vi "NovaTech409A_FreqPowPhase.vi"(2 "error in (no error)":errorcluster, 3 "Channel (0-3)":u8 max=3, 4 "Phase":u16 max=16383, 5 "Power":u16 max=1023, 6 "Freq":dbl=10.0 min=0.0 max=171.1276031, 7 "VISA resource name":refnum<visa-resource-name>="COM1") -> (0 "error out":errorcluster, 1 "VISA resource name out":refnum<visa-resource-name>="COM1")   [LabVIEW 2013, in "Novatech 409A.lvlib"]
uses:
  Novatech 409A.lvlib
panel:
  out "resulting string 3":string="P0 00000\n"
  out "read buffer 3":string
  out "resulting string 2":string="V0 0000\n"
  out "resulting string":string="F0 010.0000000\n"
  out "read buffer 2":string
  out "read buffer 1":string
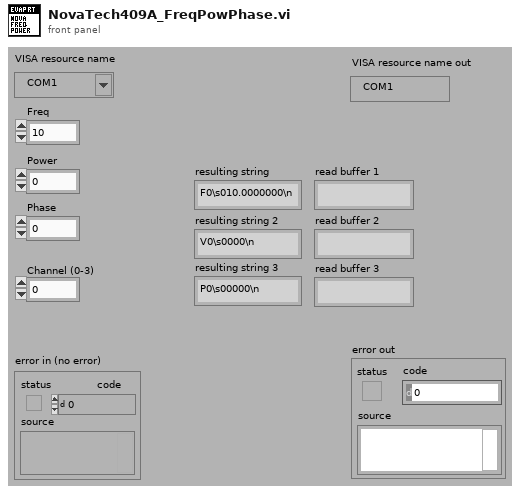
[diagram p1: front panel]
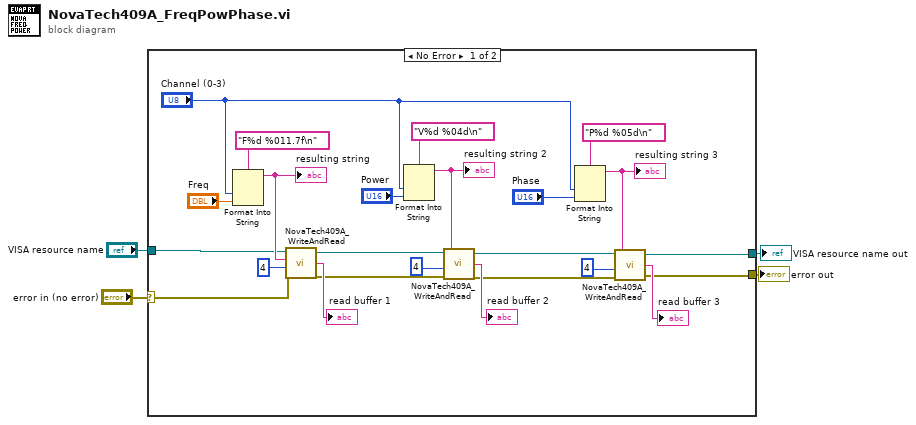
[diagram p0: block diagram]
diagram:
  n1 = case shown="No Error" "error in (no error)" {
    selector: "error in (no error)" -> [w5 w29]
    tunnel: "VISA resource name" -> [w23 w30]
    tunnel: [w7 w30] -> w3
    tunnel: [w6 w29] -> w2
    frame No Error {
      n2 = Format Into String(format string="F%d %011.7f\n", "Channel (0-3)", "Freq") -> (resulting string=w24:string)  [unwired: 2 in, 1 out]
      "resulting string" <- w24
      n3 = call "NovaTech409A_WriteAndRead.vi"("error in (no error)"=w5, "Number of Bytes"=4, "write buffer"=w24, "VISA resource name"=w23) -> ("error out"=w19:errorcluster, "read buffer"=→"read buffer 1":string, "VISA resource name out"=w20:refnum<visa-resource-name>)
      n4 = Format Into String(format string="V%d %04d\n", "Channel (0-3)", "Power") -> (resulting string=w21:string)  [unwired: 2 in, 1 out]
      "resulting string 2" <- w21
      n5 = call "NovaTech409A_WriteAndRead.vi"("error in (no error)"=w19, "Number of Bytes"=4, "write buffer"=w21, "VISA resource name"=w20) -> ("error out"=w8:errorcluster, "read buffer"=→"read buffer 2":string, "VISA resource name out"=w9:refnum<visa-resource-name>)
      n6 = Format Into String(format string="P%d %05d\n", "Channel (0-3)", "Phase") -> (resulting string=w14:string)  [unwired: 2 in, 1 out]
      "resulting string 3" <- w14
      n7 = call "NovaTech409A_WriteAndRead.vi"("error in (no error)"=w8, "Number of Bytes"=4, "write buffer"=w14, "VISA resource name"=w9) -> ("error out"=w6:errorcluster, "read buffer"=→"read buffer 3":string, "VISA resource name out"=w7:refnum<visa-resource-name>)
    }
    frame Error {
    }
  }
  "error out" <- w2
  "VISA resource name out" <- w3
